vi "AOMPowerSet.vi"(1 "AOMRelativePower":dbl) -> (0 "AOMVolts":dbl)   [LabVIEW 2017, in "SignalConverson.lvlib"]
uses:
  SignalConverson.lvlib
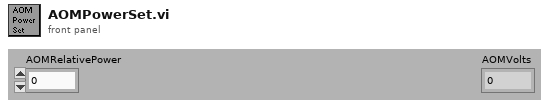
[diagram p1: front panel]
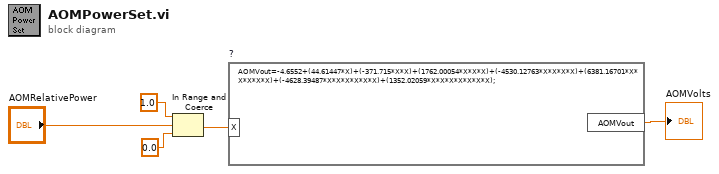
[diagram p0: block diagram]
diagram:
  n1 = In Range and Coerce(upper limit=1.0, x="AOMRelativePower", lower limit=0.0) -> (coerced(x)=w3:dbl)  [unwired: 1 out]
  n2 = formula code="AOMVout=-4.6552+(44.61447*X)+(-371.715*X*X)+(1762.00054*X*X*X)+(-4530.12763*X*X*X*X)+(6381.16701*X*X*X*X*X)+(-4628.39487*X*X*X*X*X*X)+(1352.02059*X*X*X*X*X*X*X);" "?"("X"=w3) -> ("AOMVout"=→"AOMVolts":dbl)
